vi "Check Install Error.vi"(8 "error in (no error)":errorcluster, 10 "Status in":i32, 11 "Session in":refnum<k21>) -> (0 "error out":errorcluster, 2 "Status out":i32, 3 "Session out":refnum<k21>, 4 "Details":string)   [LabVIEW 2014, in "nisyscfg.lvlib"]
uses:
  nisyscfg.lvlib
panel:
  in  "Firmware":string="Current version: %s\\nRequired version: %s\\n"
  in  "Local and Remote":string="Local file: %s\\nRemote file: %s\\n"
  in  "Remote only":string="Remote file: %s\\n"
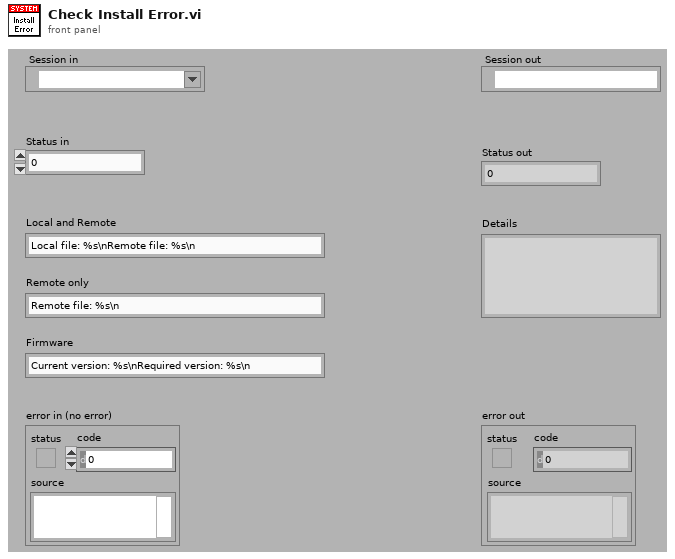
[diagram p1: front panel]
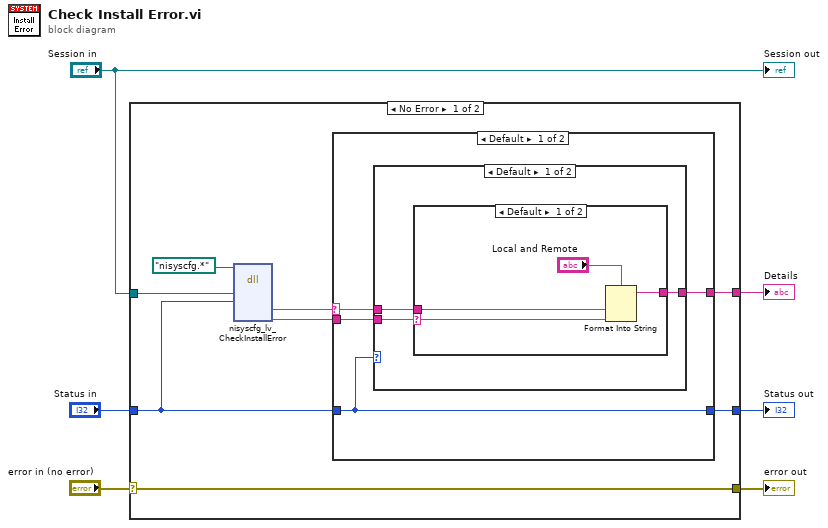
[diagram p0: block diagram]
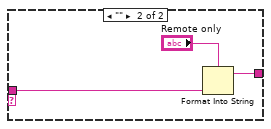
[diagram p2: hidden frame]
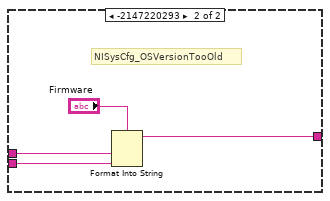
[diagram p3: hidden frame]
diagram:
  n1 = case shown="No Error" "error in (no error)" {
    selector: "error in (no error)" -> [w10 w35]
    tunnel: [w10 w35] -> w5
    tunnel: "Session in" -> [w13 _]
    tunnel: [w9 w34] -> w3
    tunnel: [w8 _] -> w2
    tunnel: "Status in" -> [w7 w34]
    frame No Error {
      n2 = dll-call lib="nisyscfg.*" fn="nisyscfg_lv_CheckInstallError" label="CheckInstallError"(path in=path "nisyscfg.*", "session"=w13, "original status"=w7) -> ("details1"=w12:string, "details2"=w11:string)  [unwired: 7 in, 2 out]
      n3 = case shown="Default" w12 {
        selector: w12 -> [w18 _]
        tunnel: w7 -> [w15 w33]
        tunnel: w11 -> [w17 _]
        tunnel: [w15 w33] -> w9
        tunnel: [w16 _] -> w8
        frame Default {
          n4 = case shown="Default" w15 {
            tunnel: w18 -> [w20 w31]
            tunnel: w17 -> [w21 w30]
            tunnel: [w19 w29] -> w16
            frame Default {
              n5 = case shown="Default" w21 {
                selector: w21 -> [w23 _]
                tunnel: w20 -> [w24 w27]
                tunnel: [w22 w26] -> w19
                frame Default {
                  n6 = Format Into String(format string="Local and Remote", w24, w23) -> (resulting string=w22:string)  [unwired: 2 in, 1 out]
                }
                frame "" {
                  n7 = Format Into String(format string="Remote only", w27) -> (resulting string=w26:string)  [unwired: 2 in, 1 out]
                }
              }
            }
            frame -2147220293 {
              # "NISysCfg_OSVersionTooOld"
              n8 = Format Into String(format string="Firmware", w31, w30) -> (resulting string=w29:string)  [unwired: 2 in, 1 out]
            }
          }
        }
        frame "" {
          # "The error was not an installation-specific code"
        }
      }
    }
    frame Error {
    }
  }
  "error out" <- w5
  "Status out" <- w3
  "Details" <- w2
  "Session out" <- "Session in"
